vi "BRig_RT__Case_Exp__State_initBlock__v17.vi"(0 "input_dataCurrent":u16[](array[numeric]), 3 "input_dataExp":u16[](array[numeric]), 4 "input_dataBlock":u16[][](array[numeric]), 5 "input_dataTrial":u16[][](array[numeric])) -> (6 "output_iSpout":u16, 7 "output_speaker_amp_R":u16, 8 "output_iBlock":u16, 9 "output_speaker_freq_R":u8, 10 "output_BUR_target":u16, 11 "output_speaker_amp_L":u16, 12 "output_TpB_target":u16, 13 "output_speaker_freq_L":u8, 14 "output_dataCurrent":u16[](array[numeric]), 18 "output_dataBlock":u16[][](array[numeric]), 19 "output_dataTrial":u16[][](array[numeric]))   [LabVIEW 2014]
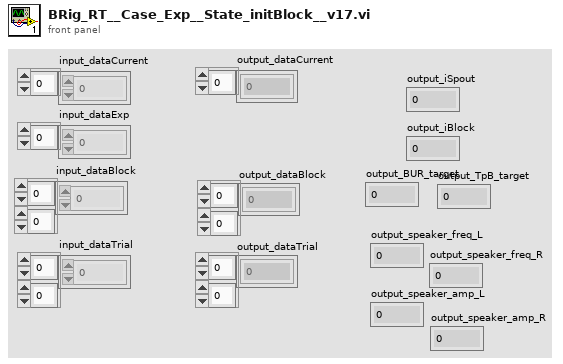
[diagram p1: front panel]
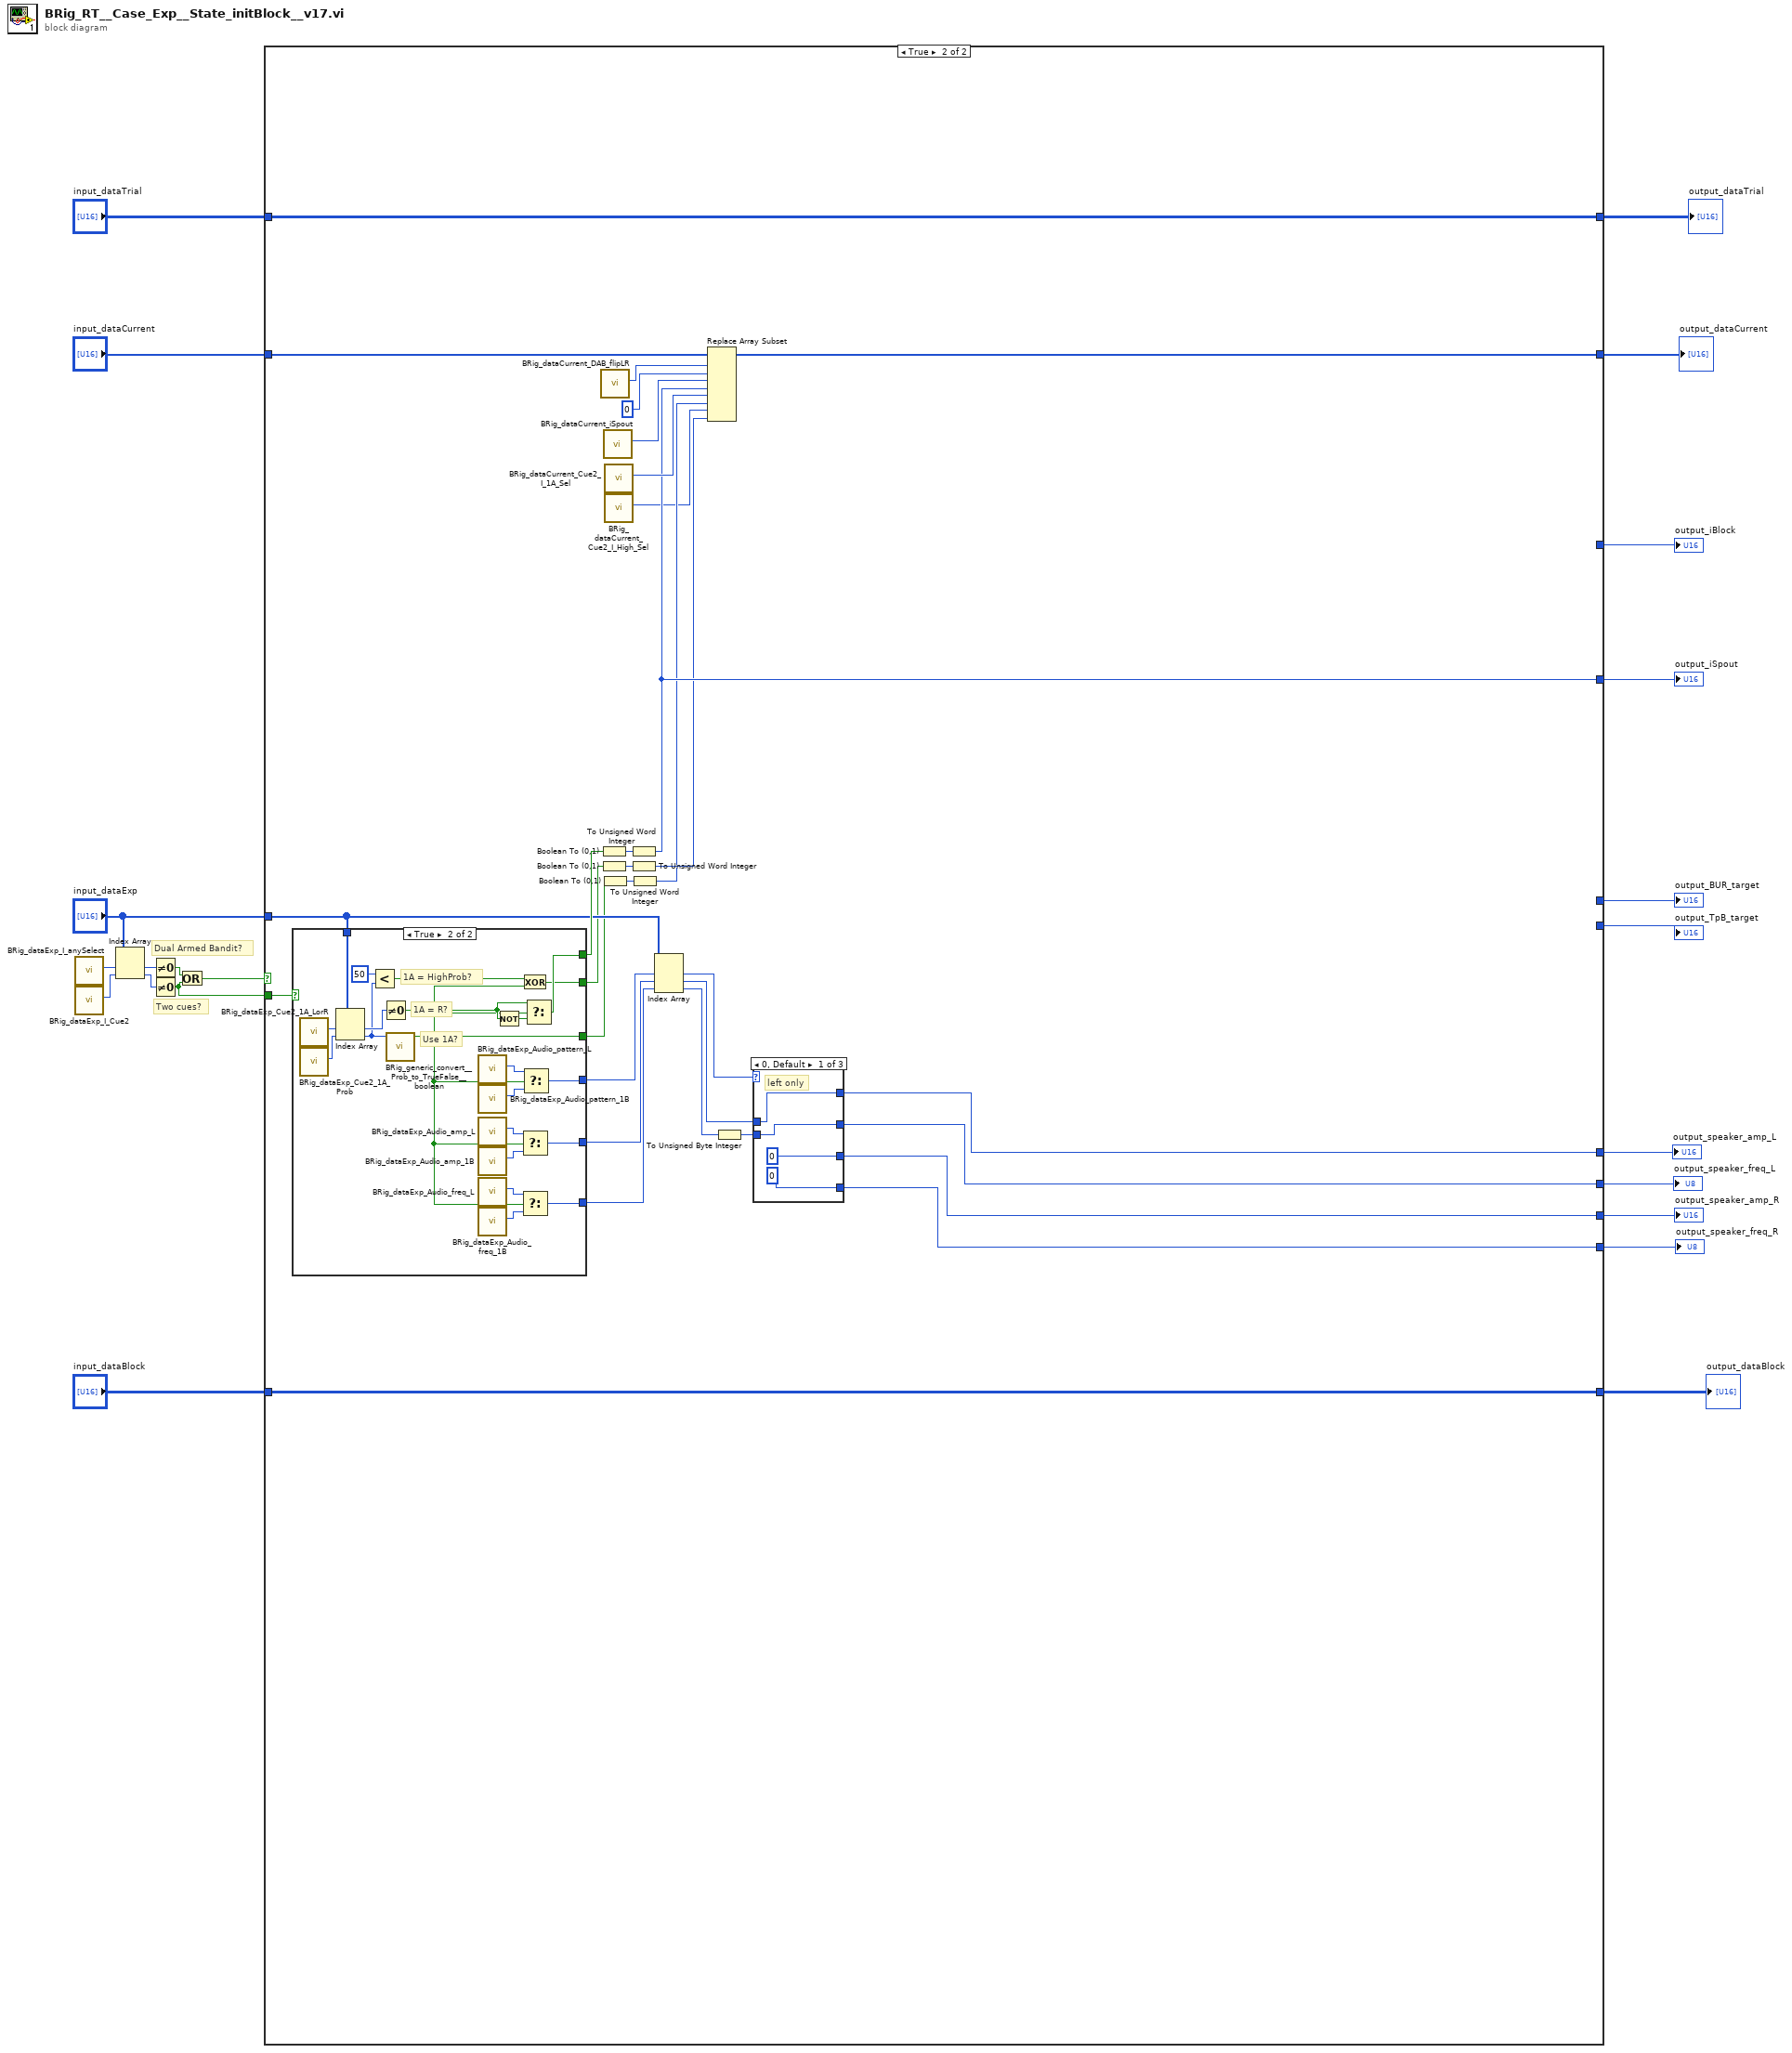
[diagram p0: block diagram]
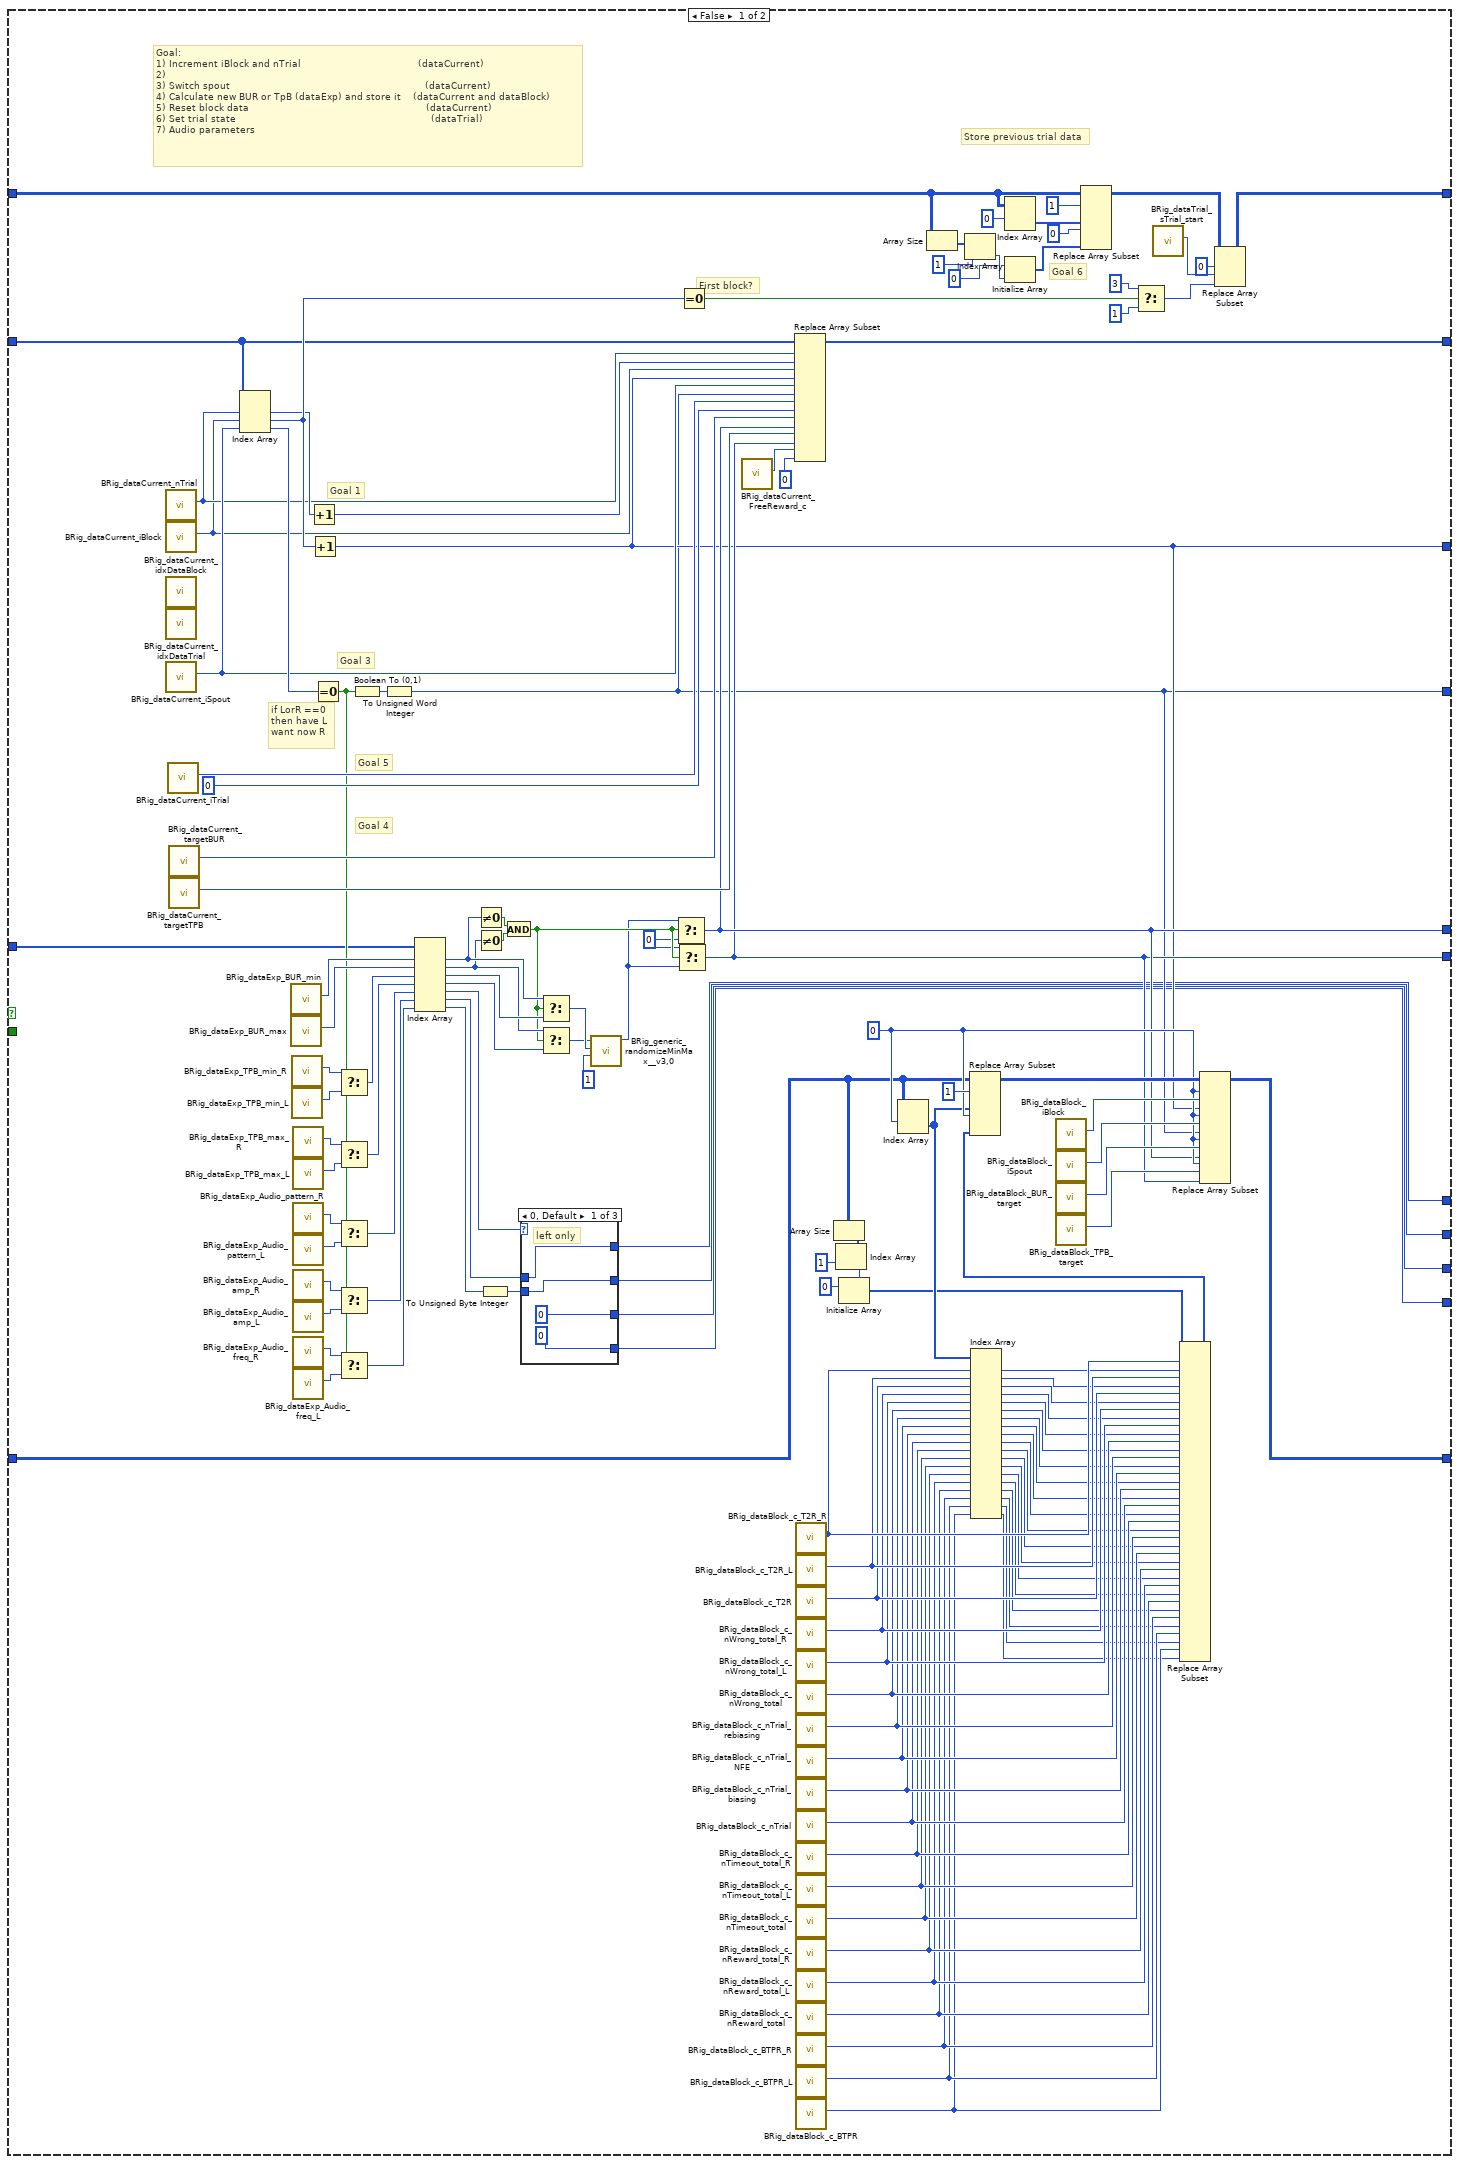
[diagram p2: hidden frame]
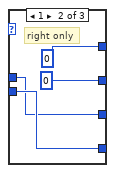
[diagram p3: hidden frame]
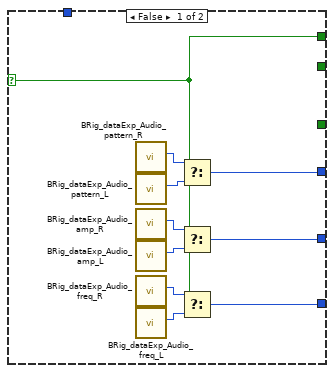
[diagram p5: hidden frame]
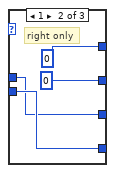
[diagram p6: hidden frame]
diagram:
  # "Two cues?"
  # "Dual Armed Bandit?"
  n1 = call "BRig_dataExp_I_anySelect.vi"() -> ("output_I_anySelect"=w21:i32)  [unwired: 11 in]
  n2 = call "BRig_dataExp_I_Cue2.vi"() -> ("output_I_Cue2"=w5:i32)  [unwired: 11 in]
  n3 = Index Array(array="input_dataExp", index #1=w21, index #2=w5) -> (element #1=w20:u16, element #2=w4:u16)
  n4 = Not Equal To 0?(x=w20) -> (x != 0?=w3:bool)
  n5 = Not Equal To 0?(x=w4) -> (x != 0?=w1:bool)
  n6 = Or(x=w3, y=w1) -> (x .or. y?=w2:bool)
  n7 = case shown="True" w2 {
    tunnel: "input_dataExp" -> [w37 w174]
    tunnel: [w36 _] -> w19
    tunnel: [w35 _] -> w18
    tunnel: [w34 _] -> w17
    tunnel: [w33 w171] -> w16
    tunnel: "input_dataBlock" -> [w32 w194]
    tunnel: [w31 w194] -> w14
    tunnel: "input_dataTrial" -> [w30 w193]
    tunnel: "input_dataCurrent" -> [w29 w183]
    tunnel: [w28 w193] -> w11
    tunnel: [w27 w182] -> w10
    tunnel: [w26 w188] -> w9
    tunnel: [w25 w187] -> w8
    tunnel: [w24 w186] -> w7
    tunnel: [w23 w185] -> w6
    tunnel: w1 -> [_ w179]
    frame False {
      w79 = 0 ("disabled index (row)")
      w135 = u16 0 ("f")
      # "Store previous trial data"
      # "if LorR ==0\nthen have L\nwant now R"
      # "First block?"
      # "Goal 6"
      # "Goal 4"
      # "Goal 5"
      # "Goal 3"
      # "Goal 1"
      # "Goal:\n1) Increment iBlock and nTrial                                       (dataCurrent)\n2) \n3) Switch spout                                                                 (dataCurrent)\n4) Calculate new BUR or TpB (dataExp) and store it    (dataCurrent and dataBlock)\n5) Reset block data                                                           (dataCurrent)\n6) Set trial state                                                                 (dataTrial)\n7) Audio parameters"
      n8 = call "BRig_dataCurrent_nTrial.vi"() -> ("output_nTrial"=w98:i32)  [unwired: 11 in]
      n9 = call "BRig_dataCurrent_iBlock.vi"() -> ("output_iBlock"=w96:i32)  [unwired: 11 in]
      n10 = call "BRig_dataCurrent_idxDataBlock.vi"() -> ()  [unwired: 11 in, 1 out]
      n11 = call "BRig_dataCurrent_idxDataTrial.vi"() -> ()  [unwired: 11 in, 1 out]
      n12 = call "BRig_dataCurrent_iSpout.vi"() -> ("output_iSpout"=w120:i32)  [unwired: 11 in]
      n13 = call "BRig_dataCurrent_iTrial.vi"() -> ("output_iTrial"=w121:i32)  [unwired: 11 in]
      n14 = call "BRig_dataCurrent_targetBUR.vi"() -> ("output_targetBUR"=w123:i32)  [unwired: 11 in]
      n15 = call "BRig_dataCurrent_targetTPB.vi"() -> ("output_targetTPB"=w124:i32)  [unwired: 11 in]
      n16 = Index Array(array=w29, index #1=w98, index #2=w96, index #3=w120) -> (element #1=w119:u16, element #2=w129:u16, element #3=w152:u16)
      n17 = call "BRig_dataExp_BUR_min.vi"() -> ("output_BUR_min"=w151:i32)  [unwired: 11 in]
      n18 = call "BRig_dataExp_BUR_max.vi"() -> ("output_BUR_max"=w150:i32)  [unwired: 11 in]
      n19 = call "BRig_dataExp_TPB_min_R.vi"() -> ("output_TPB_min_R"=w147:i32)  [unwired: 11 in]
      n20 = call "BRig_dataExp_TPB_min_L.vi"() -> ("output_TPB_min_L"=w146:i32)  [unwired: 11 in]
      n21 = call "BRig_dataExp_TPB_max_R.vi"() -> ("output_TPB_max_R"=w101:i32)  [unwired: 11 in]
      n22 = call "BRig_dataExp_TPB_max_L.vi"() -> ("output_TPB_max_L"=w100:i32)  [unwired: 11 in]
      n23 = call "BRig_dataExp_Audio_pattern_R.vi"() -> ("output_Audio_sp__R"=w117:i32)  [unwired: 11 in]
      n24 = call "BRig_dataExp_Audio_pattern_L.vi"() -> ("output_Audio_sp__L"=w116:i32)  [unwired: 11 in]
      n25 = call "BRig_dataExp_Audio_amp_R.vi"() -> ("output_Audio_amp__R"=w115:i32)  [unwired: 11 in]
      n26 = call "BRig_dataExp_Audio_amp_L.vi"() -> ("output_Audio_amp__L"=w114:i32)  [unwired: 11 in]
      n27 = call "BRig_dataExp_Audio_freq_R.vi"() -> ("output_Audio_freq__R"=w113:i32)  [unwired: 11 in]
      n28 = call "BRig_dataExp_Audio_freq_L.vi"() -> ("output_Audio_freq__L"=w112:i32)  [unwired: 11 in]
      n29 = Increment(x=w119) -> (x+1=w97:u16)
      n30 = Increment(x=w129) -> (x+1=w34:u16)
      n31 = Equal To 0?(x=w152) -> (x = 0?=w118:bool)
      n32 = Select(t=w147, s=w118, f=w146) -> (s? t:f=w145:i32)
      n33 = Select(t=w101, s=w118, f=w100) -> (s? t:f=w144:i32)
      n34 = Select(t=w117, s=w118, f=w116) -> (s? t:f=w111:i32)
      n35 = Select(t=w115, s=w118, f=w114) -> (s? t:f=w110:i32)
      n36 = Select(t=w113, s=w118, f=w112) -> (s? t:f=w109:i32)
      n37 = Boolean To (0,1)(Boolean=w118) -> (0, 1=w153:i16)
      n38 = To Unsigned Word Integer(number=w153) -> (unsigned 16bit integer=w33:u16)
      n39 = Index Array(array=w37, index #1=w151, index #2=w150, index #3=w145, index #4=w144, index #5=w111, index #6=w110, index #7=w109) -> (element #1=w143:u16, element #2=w141:u16, element #3=w142:u16, element #4=w140:u16, element #5=w108:u16, element #6=w107:u16, element #7=w106:u16)
      n40 = Not Equal To 0?(x=w143) -> (x != 0?=w148:bool)
      n41 = Not Equal To 0?(x=w141) -> (x != 0?=w149:bool)
      n42 = To Unsigned Byte Integer(number=w106) -> (unsigned 8bit integer=w105:u8)
      n43 = And(x=w148, y=w149) -> (x .and. y?=w136:bool)
      n44 = case shown="0, Default" w108 {
        tunnel: w107 -> [w157 w160 w162]
        tunnel: w105 -> [w156 w161 w163]
        tunnel: [w157 u16 0 ("Numeric") w162] -> w26
        tunnel: [w156 u8 0 w163] -> w25
        tunnel: [u8 0 w161 w163] -> w23
        tunnel: [u16 0 ("Numeric") w160 w162] -> w24
        frame 0, Default {
          # "left only"
        }
        frame 1 {
          # "right only"
        }
        frame 2 {
          # "left and right"
        }
      }
      n45 = Select(t=w143, s=w136, f=w142) -> (s? t:f=w138:u16)
      n46 = Select(t=w141, s=w136, f=w140) -> (s? t:f=w137:u16)
      n47 = call "BRig_generic_randomizeMinMax__v3,0.vi"("Input_Increment"=u16 1, "Input_Min"=w138, "Input_Max"=w137) -> ("Output"=w134:u16)  [unwired: 8 in]
      n48 = Select(t=w134, s=w136, f=w135) -> (s? t:f=w36:u16)
      n49 = Select(t=w135, s=w136, f=w134) -> (s? t:f=w35:u16)
      n50 = Equal To 0?(x=w129) -> (x = 0?=w104:bool)
      n51 = call "BRig_dataCurrent_FreeReward_c.vi"() -> ("output_FreeReward_c"=w103:i32)  [unwired: 11 in]
      n52 = Replace Array Subset(array=w29, new element #1=w97, index #1=w98, new element #2=w34, index #2=w96, new element #3=w33, index #3=w120, new element #4=u16 0 ("new element/subarray"), index #4=w121, new element #5=w36, index #5=w123, new element #6=w35, index #6=w124, new element #7=u16 0 ("new element/subarray"), index #7=w103) -> (w27:u16[])
      n53 = call "BRig_dataBlock_c_T2R_R.vi"() -> ("output_c_T2R_R"=w75:i32)  [unwired: 11 in]
      n54 = call "BRig_dataBlock_c_T2R_L.vi"() -> ("output_c_T2R_L"=w74:i32)  [unwired: 11 in]
      n55 = call "BRig_dataBlock_c_T2R.vi"() -> ("output_c_T2R"=w73:i32)  [unwired: 11 in]
      n56 = call "BRig_dataBlock_c_nWrong_total_R.vi"() -> ("output_c_nWrong_total_R"=w72:i32)  [unwired: 11 in]
      n57 = call "BRig_dataBlock_c_nWrong_total_L.vi"() -> ("output_c_nWrong_total_L"=w71:i32)  [unwired: 11 in]
      n58 = call "BRig_dataBlock_c_nWrong_total.vi"() -> ("output_c_nWrong_total"=w70:i32)  [unwired: 11 in]
      n59 = call "BRig_dataBlock_c_nTrial_rebiasing.vi"() -> ("output_c_nTrial_rebiasing"=w69:i32)  [unwired: 11 in]
      n60 = call "BRig_dataBlock_c_nTrial_NFE.vi"() -> ("output_c_nTrial_NFE"=w68:i32)  [unwired: 11 in]
      n61 = call "BRig_dataBlock_c_nTrial_biasing.vi"() -> ("output_c_nTrial_biasing"=w67:i32)  [unwired: 11 in]
      n62 = call "BRig_dataBlock_c_nTrial.vi"() -> ("output_c_nTrial"=w66:i32)  [unwired: 11 in]
      n63 = call "BRig_dataBlock_c_nTimeout_total_R.vi"() -> ("output_c_nTimeout_total_R"=w65:i32)  [unwired: 11 in]
      n64 = call "BRig_dataBlock_c_nTimeout_total_L.vi"() -> ("output_c_nTimeout_total_L"=w64:i32)  [unwired: 11 in]
      n65 = call "BRig_dataBlock_c_nTimeout_total.vi"() -> ("output_c_nTimeout_total"=w63:i32)  [unwired: 11 in]
      n66 = call "BRig_dataBlock_c_nReward_total_R.vi"() -> ("output_nReward_total_R"=w62:i32)  [unwired: 11 in]
      n67 = call "BRig_dataBlock_c_nReward_total_L.vi"() -> ("output_nReward_total_L"=w61:i32)  [unwired: 11 in]
      n68 = call "BRig_dataBlock_c_nReward_total.vi"() -> ("output_nReward_total"=w60:i32)  [unwired: 11 in]
      n69 = call "BRig_dataBlock_c_BTPR_R.vi"() -> ("output_c_BTPR_R"=w59:i32)  [unwired: 11 in]
      n70 = call "BRig_dataBlock_c_BTPR_L.vi"() -> ("output_c_BTPR_L"=w58:i32)  [unwired: 11 in]
      n71 = call "BRig_dataBlock_c_BTPR.vi"() -> ("output_c_BTPR"=w57:i32)  [unwired: 11 in]
      n72 = Array Size(array=w32) -> (size(s)=w85:i32[])
      n73 = Index Array(array=w85, index=1) -> (element=w83:i32)
      n74 = Initialize Array(u16 0 ("index"), w83) -> (w77:u16[])
      n75 = Index Array(array=w32, index (row)=w79) -> (element=w78:u16[])  [unwired: 1 in]
      n76 = Array Size(array=w30) -> (size(s)=w90:i32[])
      n77 = Index Array(array=w90, index=1) -> (element=w88:i32)
      n78 = Index Array(array=w78, index #1=w75, index #2=w74, index #3=w73, index #4=w72, index #5=w71, index #6=w70, index #7=w69, index #8=w68, index #9=w67, index #10=w66, index #11=w65, index #12=w64, index #13=w63, index #14=w62, index #15=w61, index #16=w60, index #17=w59, index #18=w58, index #19=w57) -> (element #1=w38:u16, element #2=w39:u16, element #3=w40:u16, element #4=w41:u16, element #5=w42:u16, element #6=w43:u16, element #7=w44:u16, element #8=w45:u16, element #9=w46:u16, element #10=w47:u16, element #11=w48:u16, element #12=w49:u16, element #13=w50:u16, element #14=w51:u16, element #15=w52:u16, element #16=w53:u16, element #17=w54:u16, element #18=w55:u16, element #19=w56:u16)
      n79 = Index Array(array=w30, index (row)=0) -> (element=w92:u16[])  [unwired: 1 in]
      n80 = Initialize Array(u16 0 ("index"), w88) -> (w86:u16[])
      n81 = call "BRig_dataBlock_iBlock.vi"() -> ("output_iBlock"=w133:i32)  [unwired: 11 in]
      n82 = call "BRig_dataBlock_iSpout.vi"() -> ("output_iSpout"=w132:i32)  [unwired: 11 in]
      n83 = call "BRig_dataBlock_BUR_target.vi"() -> ("output_BUR_target"=w131:i32)  [unwired: 11 in]
      n84 = call "BRig_dataBlock_TPB_target.vi"() -> ("output_TPB_target"=w130:i32)  [unwired: 11 in]
      n85 = Replace Array Subset(array=w30, new element #1=w92, index (row) #1=1 ("index (row)"), new element #2=w86, index (row) #2=0 ("index (row)")) -> (w95:u16[][])  [unwired: 2 in]
      n86 = Select(t=u16 3 ("new element/subarray"), s=w104, f=u16 1 ("new element/subarray")) -> (s? t:f=w127:u16)
      n87 = call "BRig_dataTrial_sTrial_start.vi"() -> ("output_sTrial_start"=w128:i32)  [unwired: 11 in]
      n88 = Replace Array Subset(array=w77, new element #1=w38, index #1=w75, new element #2=w39, index #2=w74, new element #3=w40, index #3=w73, new element #4=w41, index #4=w72, new element #5=w42, index #5=w71, new element #6=w43, index #6=w70, new element #7=w44, index #7=w69, new element #8=w45, index #8=w68, new element #9=w46, index #9=w67, new element #10=w47, index #10=w66, new element #11=w48, index #11=w65, new element #12=w49, index #12=w64, new element #13=w50, index #13=w63, new element #14=w51, index #14=w62, new element #15=w52, index #15=w61, new element #16=w53, index #16=w60, new element #17=w54, index #17=w59, new element #18=w55, index #18=w58, new element #19=w56, index #19=w57) -> (w76:u16[])
      n89 = Replace Array Subset(array=w32, new element #1=w78, index (row) #1=1 ("index (row)"), new element #2=w76, index (row) #2=w79) -> (w80:u16[][])  [unwired: 2 in]
      n90 = Replace Array Subset(array=w80, new element #1=w34, index (row) #1=w79, index (col) #1=w133, new element #2=w33, index (row) #2=w79, index (col) #2=w132, new element #3=w36, index (row) #3=w79, index (col) #3=w131, new element #4=w35, index (row) #4=w79, index (col) #4=w130) -> (w31:u16[][])
      n91 = Replace Array Subset(array=w95, new element=w127, index (row)=0 ("disabled index (row)"), index (col)=w128) -> (w28:u16[][])
    }
    frame True {
      n92 = case shown="True" w179 {
        selector: w179 -> [w195 _]
        tunnel: [w195 w210] -> w178
        tunnel: [w198 w225] -> w177
        tunnel: [w197 w224] -> w176
        tunnel: [w196 w223] -> w175
        tunnel: w174 -> [_ w222]
        tunnel: [_ w206] -> w169
        tunnel: [_ w205] -> w166
        frame False {
          n93 = call "BRig_dataExp_Audio_pattern_R.vi"() -> ("output_Audio_sp__R"=w199:i32)  [unwired: 11 in]
          n94 = call "BRig_dataExp_Audio_pattern_L.vi"() -> ("output_Audio_sp__L"=w200:i32)  [unwired: 11 in]
          n95 = call "BRig_dataExp_Audio_amp_R.vi"() -> ("output_Audio_amp__R"=w201:i32)  [unwired: 11 in]
          n96 = call "BRig_dataExp_Audio_amp_L.vi"() -> ("output_Audio_amp__L"=w202:i32)  [unwired: 11 in]
          n97 = call "BRig_dataExp_Audio_freq_R.vi"() -> ("output_Audio_freq__R"=w203:i32)  [unwired: 11 in]
          n98 = call "BRig_dataExp_Audio_freq_L.vi"() -> ("output_Audio_freq__L"=w204:i32)  [unwired: 11 in]
          n99 = Select(t=w199, s=w195, f=w200) -> (s? t:f=w198:i32)
          n100 = Select(t=w201, s=w195, f=w202) -> (s? t:f=w197:i32)
          n101 = Select(t=w203, s=w195, f=w204) -> (s? t:f=w196:i32)
        }
        frame True {
          # "1A = HighProb?"
          # "1A = R?"
          # "Use 1A?"
          n102 = call "BRig_dataExp_Cue2_1A_LorR.vi"() -> ("output_Cue2_1A_LorR"=w220:i32)  [unwired: 11 in]
          n103 = call "BRig_dataExp_Cue2_1A_Prob.vi"() -> ("output_Cue2_1A_Prob"=w221:i32)  [unwired: 11 in]
          n104 = Index Array(array=w222, index #1=w220, index #2=w221) -> (element #1=w213:u16, element #2=w209:u16)
          n105 = Less?(x=u16 50, y=w209) -> (x < y?=w207:bool)
          n106 = Not Equal To 0?(x=w213) -> (x != 0?=w211:bool)
          n107 = call "BRig_generic_convert__Prob_to_TrueFalse__boolean.vi"("input_probability_u16"=w209) -> ("output_TF"=w205:bool)  [unwired: 10 in]
          n108 = call "BRig_dataExp_Audio_pattern_L.vi"() -> ("output_Audio_sp__L"=w218:i32)  [unwired: 11 in]
          n109 = call "BRig_dataExp_Audio_pattern_1B.vi"() -> ("output_Audio_sp__1B"=w219:i32)  [unwired: 11 in]
          n110 = call "BRig_dataExp_Audio_amp_L.vi"() -> ("output_Audio_amp__L"=w216:i32)  [unwired: 11 in]
          n111 = call "BRig_dataExp_Audio_amp_1B.vi"() -> ("output_Audio_amp__1B"=w217:i32)  [unwired: 11 in]
          n112 = call "BRig_dataExp_Audio_freq_L.vi"() -> ("output_Audio_freq__L"=w214:i32)  [unwired: 11 in]
          n113 = call "BRig_dataExp_Audio_freq_1B.vi"() -> ("output_Audio_freq__1B"=w215:i32)  [unwired: 11 in]
          n114 = Not(x=w211) -> (.not. x?=w212:bool)
          n115 = Exclusive Or(1:w205, 2:w207) -> (0:w206:bool)
          n116 = Select(t=w216, s=w205, f=w217) -> (s? t:f=w224:i32)
          n117 = Select(t=w214, s=w205, f=w215) -> (s? t:f=w223:i32)
          n118 = Select(t=w218, s=w205, f=w219) -> (s? t:f=w225:i32)
          n119 = Select(t=w211, s=w205, f=w212) -> (s? t:f=w210:bool)
        }
      }
      n120 = Boolean To (0,1)(Boolean=w178) -> (0, 1=w184:i16)
      n121 = Boolean To (0,1)(Boolean=w169) -> (0, 1=w170:i16)
      n122 = call "BRig_dataCurrent_DAB_flipLR.vi"() -> ("output_DAB_flipLR"=w181:i32)  [unwired: 11 in]
      n123 = Boolean To (0,1)(Boolean=w166) -> (0, 1=w167:i16)
      n124 = call "BRig_dataCurrent_iSpout.vi"() -> ("output_iSpout"=w173:i32)  [unwired: 11 in]
      n125 = call "BRig_dataCurrent_Cue2_I_1A_Sel.vi"() -> ("output_Cue2_I_1A_Sel"=w172:i32)  [unwired: 11 in]
      n126 = call "BRig_dataCurrent_Cue2_I_High_Sel.vi"() -> ("output_Cue2_I_High_Sel"=w164:i32)  [unwired: 11 in]
      n127 = To Unsigned Word Integer(number=w184) -> (unsigned 16bit integer=w171:u16)
      n128 = To Unsigned Word Integer(number=w170) -> (unsigned 16bit integer=w168:u16)
      n129 = To Unsigned Word Integer(number=w167) -> (unsigned 16bit integer=w165:u16)
      n130 = Index Array(array=w174, index #1=w177, index #2=w176, index #3=w175) -> (element #1=w192:u16, element #2=w191:u16, element #3=w190:u16)
      n131 = Replace Array Subset(array=w183, new element #1=u16 0 ("new element/subarray"), index #1=w181, new element #2=w171, index #2=w173, new element #3=w165, index #3=w172, new element #4=w168, index #4=w164) -> (w182:u16[])
      n132 = To Unsigned Byte Integer(number=w190) -> (unsigned 8bit integer=w189:u8)
      n133 = case shown="0, Default" w192 {
        tunnel: w191 -> [w229 w232 w234]
        tunnel: w189 -> [w228 w233 w235]
        tunnel: [w229 u16 0 ("Numeric") w234] -> w188
        tunnel: [w228 u8 0 w235] -> w187
        tunnel: [u8 0 w233 w235] -> w185
        tunnel: [u16 0 ("Numeric") w232 w234] -> w186
        frame 0, Default {
          # "left only"
        }
        frame 1 {
          # "right only"
        }
        frame 2 {
          # "left and right"
        }
      }
    }
  }
  "output_BUR_target" <- w19
  "output_TpB_target" <- w18
  "output_iBlock" <- w17
  "output_iSpout" <- w16
  "output_dataBlock" <- w14
  "output_dataTrial" <- w11
  "output_dataCurrent" <- w10
  "output_speaker_amp_L" <- w9
  "output_speaker_freq_L" <- w8
  "output_speaker_amp_R" <- w7
  "output_speaker_freq_R" <- w6
